vi "MQTT_Q_PVT_GetSetConnRef.vi"(6 "IsReadOnlyConn?":bool, 7 "Set?":bool, 8 "error in (no error)":errorcluster, 10 "connection ID In":refnum<k5>, 11 "MQTT_Q in":refnum<class "MQTT_Q.lvclass">) -> (0 "error out":errorcluster, 2 "connection ID Out":refnum<k5>, 3 "MQTT_Q out":refnum<class "MQTT_Q.lvclass">)   [LabVIEW 2015, in "MQTT_Q.lvclass"]
uses:
  MQTT_Q.lvclass
  MQTT_Q.lvclass/MQTT_Q.ctl
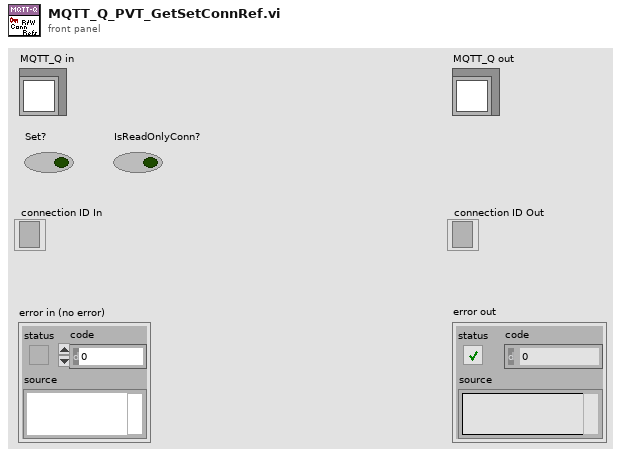
[diagram p1: front panel]
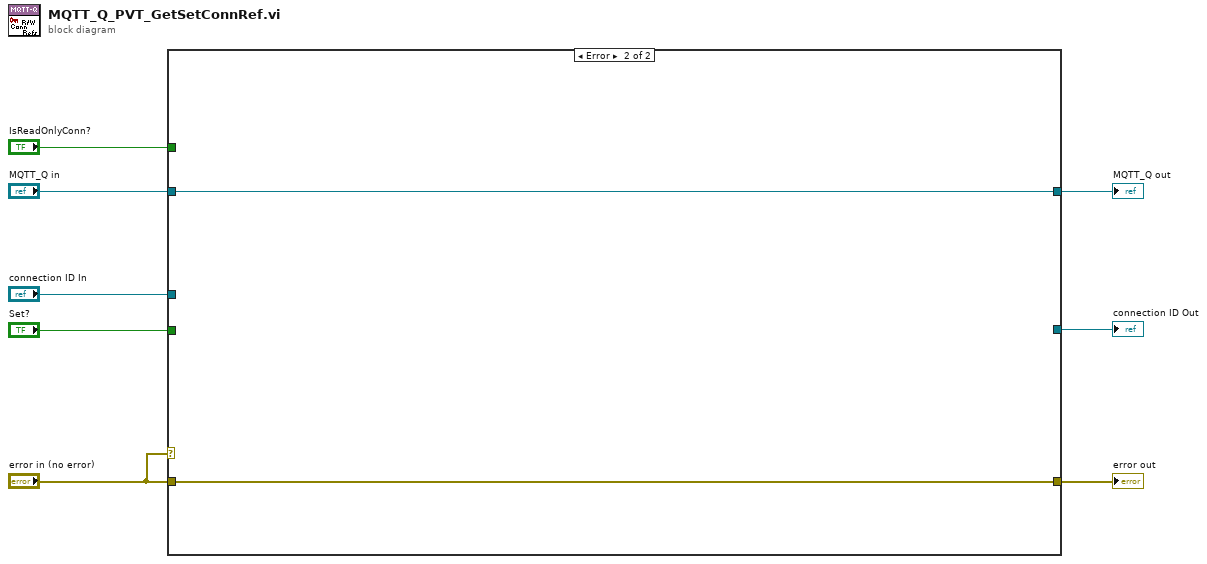
[diagram p0: block diagram]
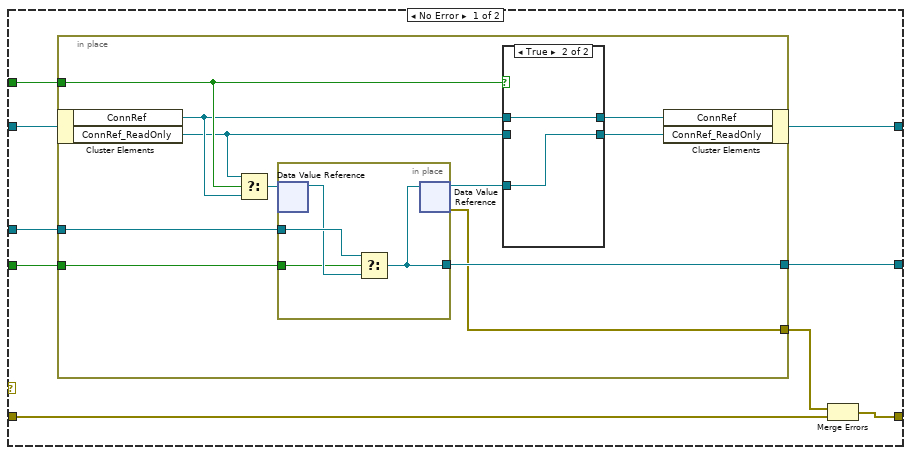
[diagram p2: hidden frame]
diagram:
  n1 = case shown="Error" "error in (no error)" {
    tunnel: "MQTT_Q in" -> [w17 w37]
    tunnel: [w16 w37] -> w7
    tunnel: "Set?" -> [w15 _]
    tunnel: "connection ID In" -> [w14 _]
    tunnel: [w13 _] -> w4
    tunnel: "error in (no error)" -> [w11 w38]
    tunnel: [w10 w38] -> w3
    tunnel: "IsReadOnlyConn?" -> [w9 _]
    frame No Error {
      n2 = in-place {
        in-place-border: w15 -> [w28]
        in-place-border: w14 -> [w27]
        in-place-border: [w26] -> w13
        in-place-border: [w25] -> w12
        in-place-border: w9 -> [w23]
        n3 = in-place-cluster #1(w17) -> ("ConnRef"=w19:refnum<data-value>, "ConnRef_ReadOnly"=w18:refnum<data-value>)
        n4 = Select(t=w18, s=w23, f=w19) -> (s? t:f=w24:refnum<data-value>)
        n5 = in-place {
          in-place-border: w28 -> [w33]
          in-place-border: w27 -> [w36]
          in-place-border: [w34] -> w26
          n6 = in-place-dvr #2(w24) -> (w35:refnum<k5>)  [unwired: 1 out]
          n7 = Select(t=w36, s=w33, f=w35) -> (s? t:f=w34:refnum<k5>)
          n8 = in-place-dvr #2(w34) -> (w22:refnum<data-value>, w25:errorcluster)
        }
        n9 = case shown="True" w23 {
          tunnel: w22 -> [w30 w32]
          tunnel: [w29 w32] -> w21
          tunnel: [w30 w31] -> w20
          tunnel: w19 -> [_ w31]
          tunnel: w18 -> [w29 _]
          frame False {
          }
          frame True {
          }
        }
        n10 = in-place-cluster #1("ConnRef"=w20, "ConnRef_ReadOnly"=w21) -> (w16:refnum<class "MQTT_Q.lvclass">)
      }
      n11 = Merge Errors(w12, w11) -> (w10:errorcluster)
    }
    frame Error {
    }
  }
  "error out" <- w3
  "MQTT_Q out" <- w7
  "connection ID Out" <- w4
